vi "Unpack.vi"(8 "error in":errorcluster, 10 "destination folder":path, 11 "nipkg filepath":path) -> (0 "error out":errorcluster)   [LabVIEW 2014, in "NIPM_API.lvlib"]
doc: "Unpacks an existing package"
uses:
  NIPM_API.lvlib
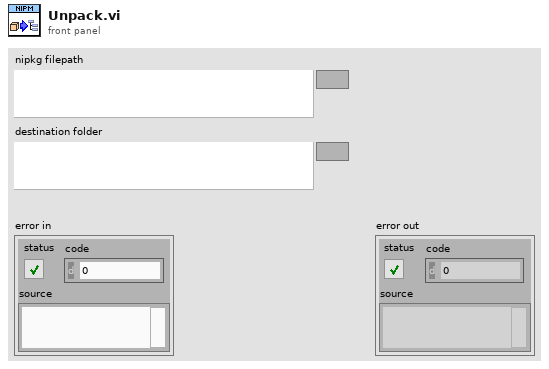
[diagram p1: front panel]
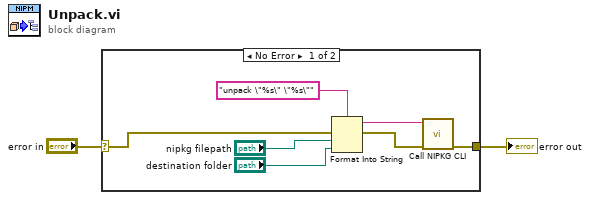
[diagram p0: block diagram]
diagram:
  n1 = case shown="No Error" "error in" {
    selector: "error in" -> [w6 w10]
    tunnel: [w3 w10] -> w1
    frame No Error {
      n2 = Format Into String(format string="unpack \"%s\" \"%s\"", error in=w6, "nipkg filepath", "destination folder") -> (resulting string=w5:string, error out=w4:errorcluster)  [unwired: 1 in]
      n3 = call "Call NIPKG CLI.vi"("error in (no error)"=w4, "command"=w5) -> ("error out"=w3:errorcluster)  [unwired: 8 in, 1 out]
    }
    frame Error {
    }
  }
  "error out" <- w1
